vi "Write VIEW.vi"(8 "error in (no error)":errorcluster, 10 "VIEW.lvclass":refnum<class "VIEW.lvclass">, 11 "CONTROLLER in":refnum<class "CONTROLLER.lvclass">) -> (0 "error out":errorcluster, 3 "CONTROLLER out":refnum<class "CONTROLLER.lvclass">)   [LabVIEW 2013, in "CONTROLLER.lvclass"]
uses:
  CONTROLLER.lvclass
  View/base/VIEW.lvclass
  CONTROLLER.lvclass/CONTROLLER.ctl
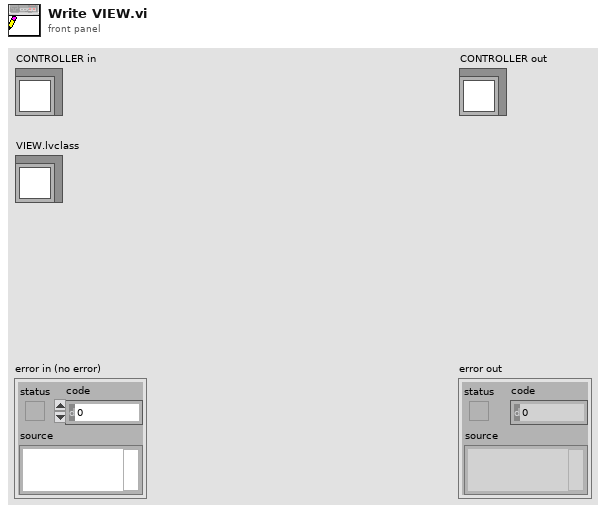
[diagram p1: front panel]
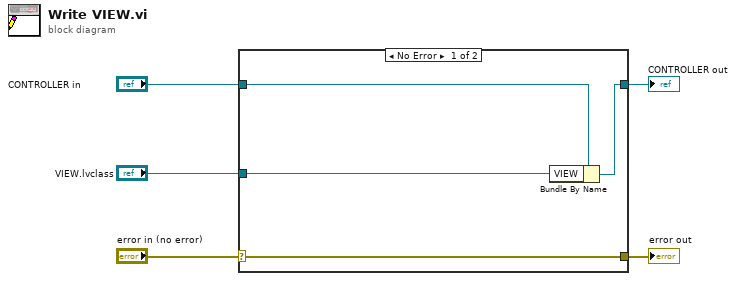
[diagram p0: block diagram]
diagram:
  n1 = case shown="No Error" "error in (no error)" {
    selector: "error in (no error)" -> [w9 w10]
    tunnel: [w9 w10] -> w4
    tunnel: [w7 w11] -> w2
    tunnel: "CONTROLLER in" -> [w8 w11]
    tunnel: "VIEW.lvclass" -> [w6 _]
    frame No Error {
      n2 = Bundle By Name(cluster=w8, "VIEW"=w6) -> (w7:refnum<class "CONTROLLER.lvclass">)
    }
    frame Error {
    }
  }
  "error out" <- w4
  "CONTROLLER out" <- w2
